vi "Blinker Text Changer.vi"(10 "In":T1=enum."Measuring") -> (2 "String Out":string)   [LabVIEW 2012]
uses:
  Control 1.ctl
  Abstract Display.lvclass
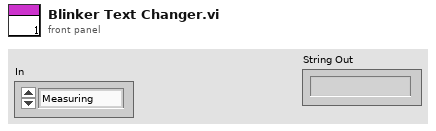
[diagram p1: front panel]
types:
  T1 = typedef "Display Panel.lvlib/Abstract Display.lvclass/Control 1.ctl" = enum16{"Done", "Warming", "Measuring"}
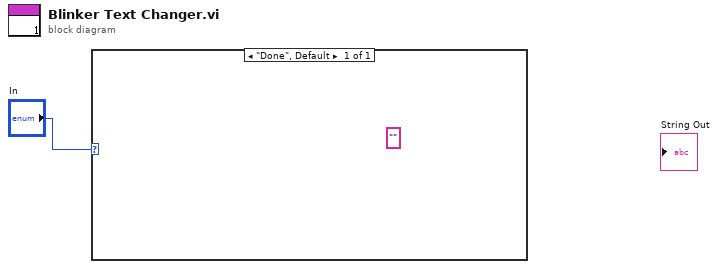
[diagram p0: block diagram]
diagram:
  n1 = case shown="\"Done\", Default" "In" {
    frame "Done", Default {
      (unwired) ""
    }
  }
